vi "v_limiter_6dof.vi"(1 "Filters":T1(array[cluster]), 3 "Sampling frequency":sgl, 4 "Reset":bool, 5 "Input":sgl[][](array[numeric]), 6 "Parameters":T2={"Stimulus"={"Type"=enum."Off", "Phase"=0.0, "Amplitude"=[], "Injection point"=enum."Total pose", "Closed loop"=FALSE, "Offset"=[], "Tip -> world"=FALSE, "Frequency"=0.0, "Length"=0.0}, "Goal Filter A"={"Speedup max"=0.0, "Speedup thresh"=0.0, "Speedup nonlin"=0.0, "Filters"=[]}, "Mode controls"={"Hold"=FALSE, "Cancellation"=FALSE, "Goal filter"=FALSE, "Trigger"=FALSE}, "Manipulator type"=enum."Current piezo", "Manipulator calibration"={"Tool offsets"=[[0.0, 0.0, 36200.0]], "Handle light calibration"=[], "Base pivots"=[], "Output pivots"=[], "Length center"=0.0, "Workspace height"=[], "Workspace diameter"=[0.0, 0.0, 36200.0], "Stack travel"=400.0, "Saturation pos"=375.0, "Inverse filters"=[], "Strut length"=0.0}, "Network"={"Remote Host"="", "Send Status"=FALSE, "Send Port"=0, "Recv Commands"=FALSE, "Recv Port"=0}, "Goal Filter B"={"Speedup max"=0.0, "Speedup thresh"=0.0, "Speedup nonlin"=0.0, "Filters"=[]}, "Cancellation"={"KP"={"XY"=0.0, "Rxy"=0.0, "Z"=0.0, "Rz"=0.0}, "KI"=0.0, "KD"={"XY"=0.0, "Rxy"=0.0, "Z"=0.0, "Rz"=0.0}, "Max vel"=20.0, "Max acc"=0.001, "Int error limit"=3.0, "RCM gain"=0.0, "Bypass"=FALSE, "Degraded gain"=0.0}, "Transition time"=0.0, "Estimation"={"Link"={"Measure noise"=[], "Process noise"=[], "Alt process noise"=[], "Alt turnoff cycles"=20, "Innovation limit"=[], "Residue threshold"=0.0, "Enable"=FALSE}, "Handle"={"Measure noise"=[], "Process noise"=[], "State limits"=[], "Innovation limit"=[], "Prediction Lookahead"=0.0, "Enable"=FALSE}}} {"Transition time" format="%_3f"; "Cancellation"."Degraded gain" min=0 max=1 step=0.1 format="%#_3p"; "Cancellation"."RCM gain" min=0 max=1 step=0.1 format="%#_3p"; "Cancellation"."KD"."Rz" min=-1 max=1 step=0.01 format="%#_3p"; "Cancellation"."KD"."Rxy" min=-1 max=1 step=0.01 format="%#_3p"; "Cancellation"."KD"."Z" min=-1 max=1 step=0.01 format="%#_3p"; "Cancellation"."KD"."XY" min=-1 max=1 step=0.01 format="%#_3p"; "Cancellation"."KI" min=0 max=1 step=0.01 format="%#_3p"; "Cancellation"."KP"."Rz" min=-1 max=1 step=0.01 format="%#_3p"; "Cancellation"."KP"."Rxy" min=-1 max=1 step=0.01 format="%#_3p"; "Cancellation"."KP"."Z" min=-1 max=1 step=0.01 format="%#_3p"; "Cancellation"."KP"."XY" min=-1 max=1 step=0.01 format="%#_3p"; "Cancellation"."Max acc" format="%#_3p"; "Goal Filter B"."Filters"."V limit range" format="%_3p"; "Goal Filter B"."Filters"."V limit" format="%_3p"; "Goal Filter B"."Filters"."Upper Q" format="%_3f"; "Goal Filter B"."Filters"."Upper Fc" format="%_3p"; "Goal Filter B"."Filters"."Lower Q" format="%_3f"; "Goal Filter B"."Filters"."Scale factor" format="%_3f"; "Goal Filter B"."Filters"."Lower Fc" format="%_3p"; "Goal Filter B"."Speedup nonlin" format="%_3p"; "Goal Filter B"."Speedup thresh" format="%_3p"; "Goal Filter B"."Speedup max" format="%_3p"; "Manipulator calibration"."Strut length" format="%#_4p"; "Manipulator calibration"."Saturation pos" format="%#.1f"; "Manipulator calibration"."Stack travel" format="%#.1f"; "Manipulator calibration"."Length center" format="%#_4p"; "Manipulator calibration"."Output pivots" format="%#_6f"; "Manipulator calibration"."Base pivots" format="%#_6f"; "Manipulator calibration"."Handle light calibration" format="%#.1f"; "Goal Filter A"."Filters"."V limit range" format="%_3p"; "Goal Filter A"."Filters"."V limit" format="%_3p"; "Goal Filter A"."Filters"."Upper Q" format="%_3f"; "Goal Filter A"."Filters"."Upper Fc" format="%_3p"; "Goal Filter A"."Filters"."Lower Q" format="%_3f"; "Goal Filter A"."Filters"."Scale factor" format="%_3f"; "Goal Filter A"."Filters"."Lower Fc" format="%_3p"; "Goal Filter A"."Speedup nonlin" format="%_3p"; "Goal Filter A"."Speedup thresh" format="%_3p"; "Goal Filter A"."Speedup max" format="%_3p"; "Stimulus"."Length" min=0.0 max=100.0 step=100.0 format="%#_4p"; "Stimulus"."Frequency" min=0.0 step=100.0 format="%#_4g"; "Stimulus"."Offset" format="%#_3p"; "Stimulus"."Amplitude" format="%#_3p"; "Stimulus"."Phase" min=-180.0 max=360.0 step=100.0 format="%#.2f"}) -> (0 "Goal position out":sgl[][](array[numeric]))   [LabVIEW 2014]
uses:
  testing/Micron params.ctl
  testing/stimulus.ctl
  testing/injection_point.ctl
  goal_loop_parms.ctl
  testing/mode_conrols.ctl
  testing/manipulator_cal.ctl
  asap/labview/testing/probe_calibration.ctl
  host/network_params.ctl
  cancellation/sq_control_params.ctl
  cancellation/decoupled_gain.ctl
  cancellation/estimation_controls.ctl
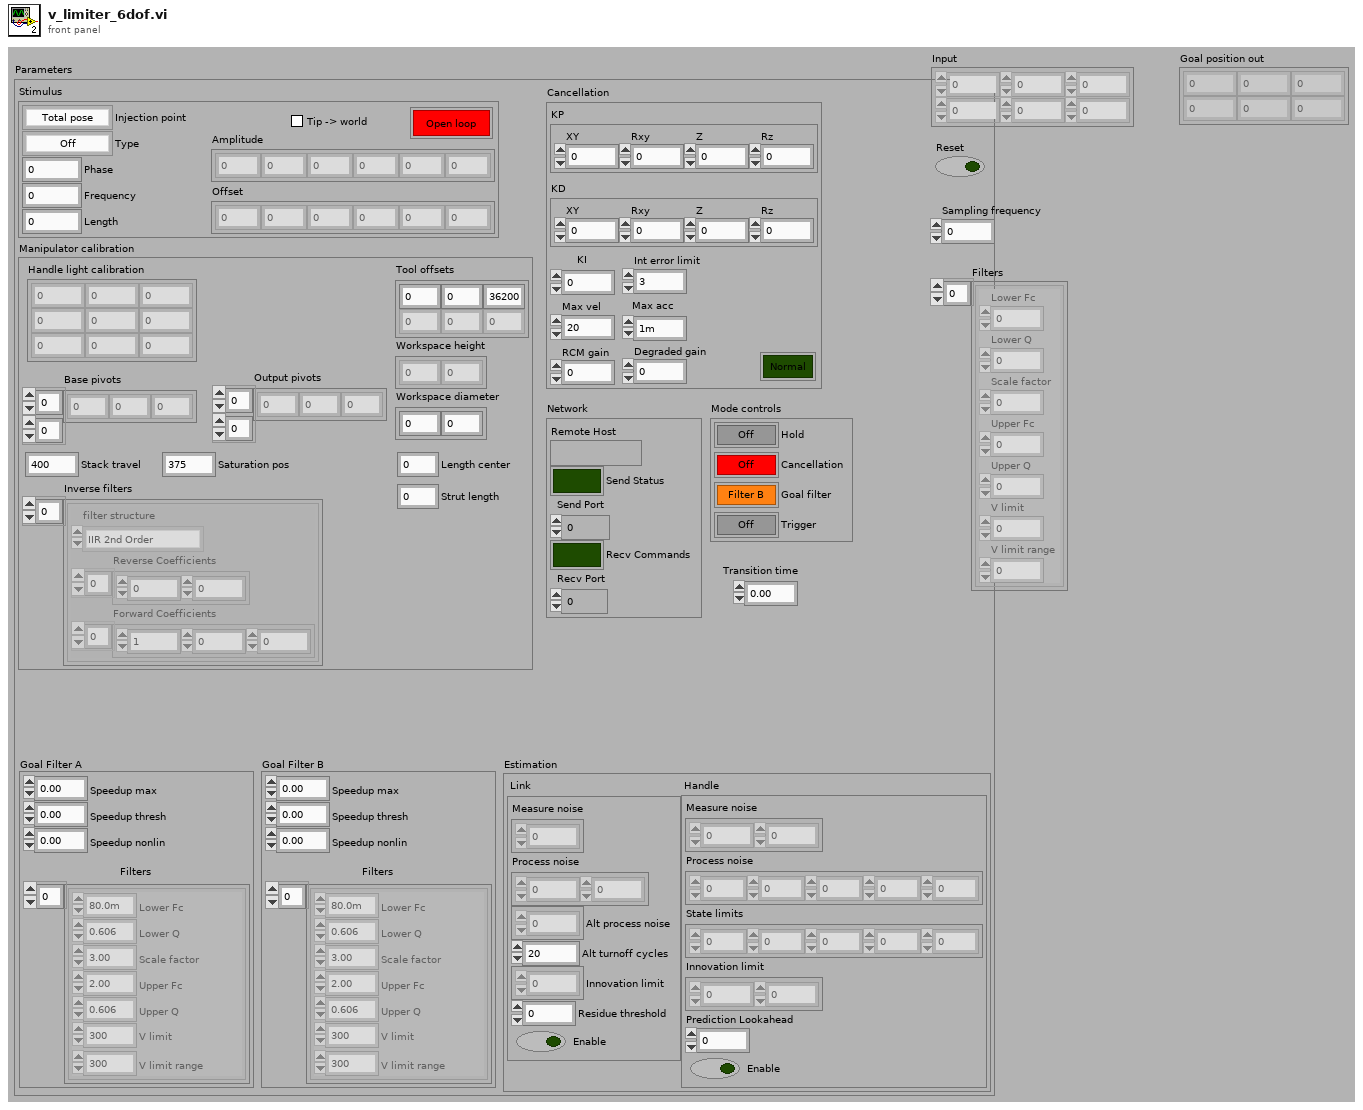
[diagram p1: front panel]
types:
  T1 = cluster{"Lower Fc":sgl, "Lower Q":sgl, "Scale factor":sgl, "Upper Fc":sgl, "Upper Q":sgl, "V limit":sgl, "V limit range":sgl}[]
  T2 = typedef "Micron params.ctl" = cluster{"Stimulus":T3, "Goal Filter A":T5, "Mode controls":T6, "Manipulator type":enum16{"Current piezo", "Voltage piezo"}, "Manipulator calibration":T7, "Network":T9, "Goal Filter B":T5, "Cancellation":T10, "Transition time":sgl, "Estimation":T12}
  T3 = typedef "stimulus.ctl" = cluster{"Type":enum16{"Off", "Step", "Sine", "Triangle", "Arbitrary"}, "Phase":dbl, "Amplitude":sgl[], "Injection point":T4, "Closed loop":bool, "Offset":sgl[], "Tip -> world":bool, "Frequency":dbl, "Length":dbl}
  T4 = typedef "injection_point.ctl" = enum16{"Total pose", "V limiter", "Goal ", "Link position", "KF link position", "Inverse kin", "Link goal", "Link error", "Controller", "Output", "Drive", "Light"}
  T5 = typedef "goal_loop_parms.ctl" = cluster{"Speedup max":sgl, "Speedup thresh":sgl, "Speedup nonlin":sgl, "Filters":cluster{"Lower Fc":sgl, "Lower Q":sgl, "Scale factor":sgl, "Upper Fc":sgl, "Upper Q":sgl, "V limit":sgl, "V limit range":sgl}[]}
  T6 = typedef "mode_conrols.ctl" = cluster{"Hold":bool, "Cancellation":bool, "Goal filter":bool, "Trigger":bool}
  T7 = typedef "manipulator_cal.ctl" = cluster{"Tool offsets":sgl[][], "Handle light calibration":T8, "Base pivots":sgl[][], "Output pivots":sgl[][], "Length center":sgl, "Workspace height":sgl[], "Workspace diameter":sgl[], "Stack travel":sgl, "Saturation pos":sgl, "Inverse filters":cluster{"filter structure":enum32{"IIR 2nd Order", "IIR 4th Order"}, "Reverse Coefficients":dbl[], "Forward Coefficients":dbl[]}[], "Strut length":sgl}
  T8 = typedef "probe_calibration.ctl" = sgl[][]
  T9 = typedef "network_params.ctl" = cluster{"Remote Host":string, "Send Status":bool, "Send Port":u16, "Recv Commands":bool, "Recv Port":u16}
  T10 = typedef "sq_control_params.ctl" = cluster{"KP":T11, "KI":sgl, "KD":T11, "Max vel":sgl, "Max acc":sgl, "Int error limit":sgl, "RCM gain":sgl, "Bypass":bool, "Degraded gain":sgl}
  T11 = typedef "decoupled_gain.ctl" = cluster{"XY":sgl, "Rxy":sgl, "Z":sgl, "Rz":sgl}
  T12 = typedef "estimation_controls.ctl" = cluster{"Link":cluster{"Measure noise":dbl[], "Process noise":dbl[], "Alt process noise":dbl[], "Alt turnoff cycles":i32, "Innovation limit":dbl[], "Residue threshold":dbl, "Enable":bool}, "Handle":cluster{"Measure noise":dbl[], "Process noise":dbl[], "State limits":dbl[], "Innovation limit":dbl[], "Prediction Lookahead":sgl, "Enable":bool}}
  T13 = cluster{"Lower Fc":sgl, "Lower Q":sgl, "Scale factor":sgl, "Upper Fc":sgl, "Upper Q":sgl, "V limit":sgl, "V limit range":sgl}
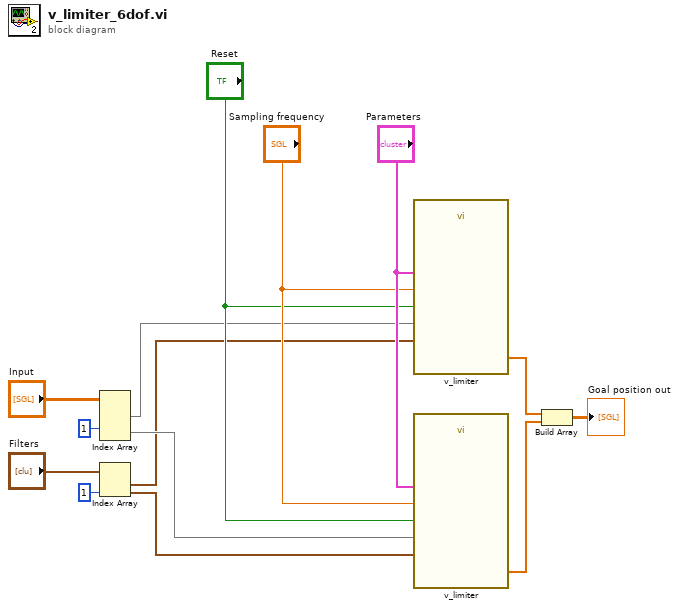
[diagram p0: block diagram]
diagram:
  n1 = Index Array(array="Input", index (row) #2=1 ("index (row)")) -> (element #1=w7:sgl[], element #2=w6:sgl[])  [unwired: 3 in]
  n2 = Index Array(array="Filters", index #2=1 ("index (row)")) -> (element #1=w5:T13, element #2=w4:T13)  [unwired: 1 in]
  n3 = call "v_limiter.vi"("Parameters"="Parameters", "Reset"="Reset", "Sampling frequency"="Sampling frequency", "Goal position in"=w7, "Goal filter"=w5) -> ("Goal position out"=w3:sgl[])  [unwired: 5 in, 1 out]
  n4 = call "v_limiter.vi"("Parameters"="Parameters", "Reset"="Reset", "Sampling frequency"="Sampling frequency", "Goal position in"=w6, "Goal filter"=w4) -> ("Goal position out"=w2:sgl[])  [unwired: 5 in, 1 out]
  n5 = Build Array(w3, w2) -> (→"Goal position out":sgl[][])
